vi "Arduino Wait for Move Complete.vi"(8 "error in (no error)":errorcluster, 11 "reference":refnum<visa-resource-name>) -> (0 "error out":errorcluster, 1 "response":string, 2 "distance":i32, 3 "Motor":i32)   [LabVIEW 2024, in "FW Arduino Control.lvclass"]
uses:
  FW Arduino Control.lvclass
  ef667a97-bf22-4261-9fe2-826bdb4b0545.vi
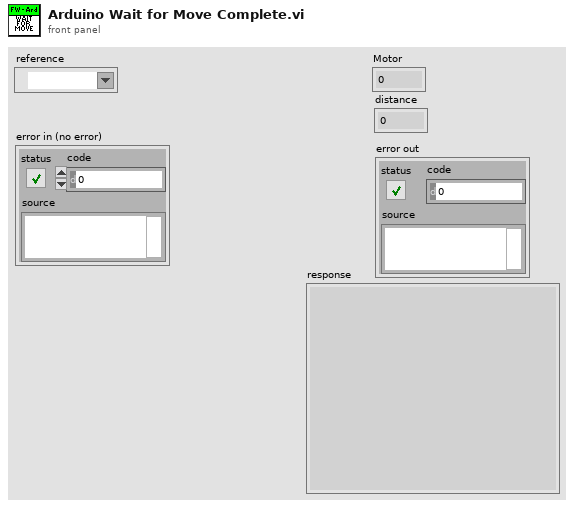
[diagram p1: front panel]
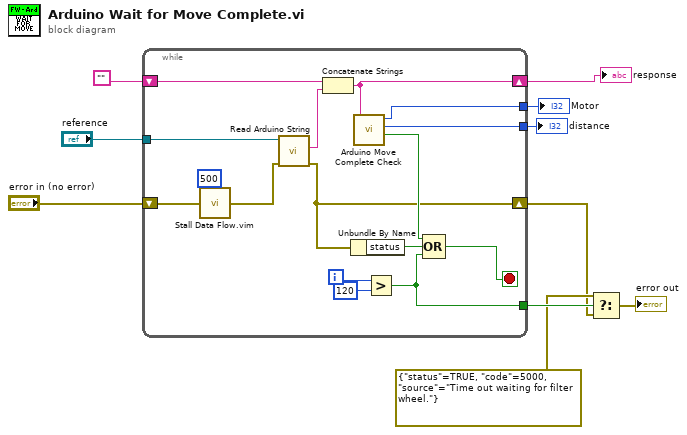
[diagram p0: block diagram]
diagram:
  n1 = while {
    tunnel: "reference" -> [w26]
    shift-right: [w15] -> w4
    shift-left: "error in (no error)" -> [w25]
    tunnel: [w20] -> w8
    tunnel: [w19] -> w7
    tunnel: [w14] -> w6
    shift-right: [w11] -> w1
    shift-left: "" -> [w13]
    i -> [w17]
    stop <- w18 stop-if-true
    n2 = call "Stall Data Flow.vim"("value in"=w25, "milliseconds to wait"=u32 500) -> ("value out"=w23:errorcluster)  [unwired: 1 out]
    n3 = call "Read Arduino String.vi"("error in (no error)"=w23, "reference"=w26) -> ("error out"=w15:errorcluster, "response"=w12:string)  [unwired: 7 in, 1 out]
    n4 = Concatenate Strings(w13, w12) -> (w11:string)
    n5 = Unbundle By Name(w15) -> ("status"=w22:bool)
    n6 = call "Arduino Move Complete Check.vi"("input string"=w11) -> ("Complete?"=w21:bool, "position"=w19:i32, "m"=w20:i32)  [unwired: 7 in, 1 out]
    n7 = Greater?(x=w17, y=120) -> (0:w14:bool)
    n8 = Compound Arithmetic op=OR(w21, w22, w14) -> (w18:bool)
  }
  "Motor" <- w8
  "distance" <- w7
  "response" <- w1
  n9 = Select(t=errorcluster {"status"=TRUE, "code"=5000, "source"="Time out waiting for filter wheel."} ("error in (no error)"), s=w6, f=w4) -> (s? t:f=→"error out":errorcluster)
